vi "Задание_АБ_расп._Рэлея.vi"() -> ()   [LabVIEW 2017]
uses:
  <vilib>/gmath/statdist.llb/Beta Random.vi
  <vilib>/Analysis/3filter.llb/Bessel Filter (DBL).vi
  <vilib>/Analysis/NI_AALBase.lvlib
  <vilib>/gmath/NI_Gmath.lvlib
panel:
  in  "Параметр масштаба":dbl=0.5 format="%#_13g"
  in  "Медиана":dbl=0.1 format="%#_13g"
  out "Шум на основе распределения Рэлея":dbl[](graph)
  out "Итого. кол-во бит":i32
  in  "Пороговое \nзначение":dbl(slide) scale=-0.5..5.0
  out "Демодулированный и отфильтрованный сигнал":dbl[][](graph)
  out "Сигнал после детектора":i16[](graph)
  in  "Нижняя частота среза":dbl
  in  "Порядок фильтра":i64(slide) scale=0.0..20.0
  in  "Переменная floor(x/y)":i32
  out "Модулирующий сигнал":dbl[](graph)
  out "Частотно модулированный цифровой сигнал":dbl[](graph)
  in  "см. 1.2 Циклов в секунду":i32(slide) scale=4.0..50.0
  in  "Сколько битов брать":i32=4
  out "Радио сигнал с паузами":dbl[](graph)
  in  "Кол-во выборок":i32=400
  out "Массив с паузами":dbl[](array[numeric])
  in  "Количество бит":i32=8
  out "Вырезка из массива":dbl[](array[numeric])
  out "Биты на выходе 1":dbl[](array[numeric])
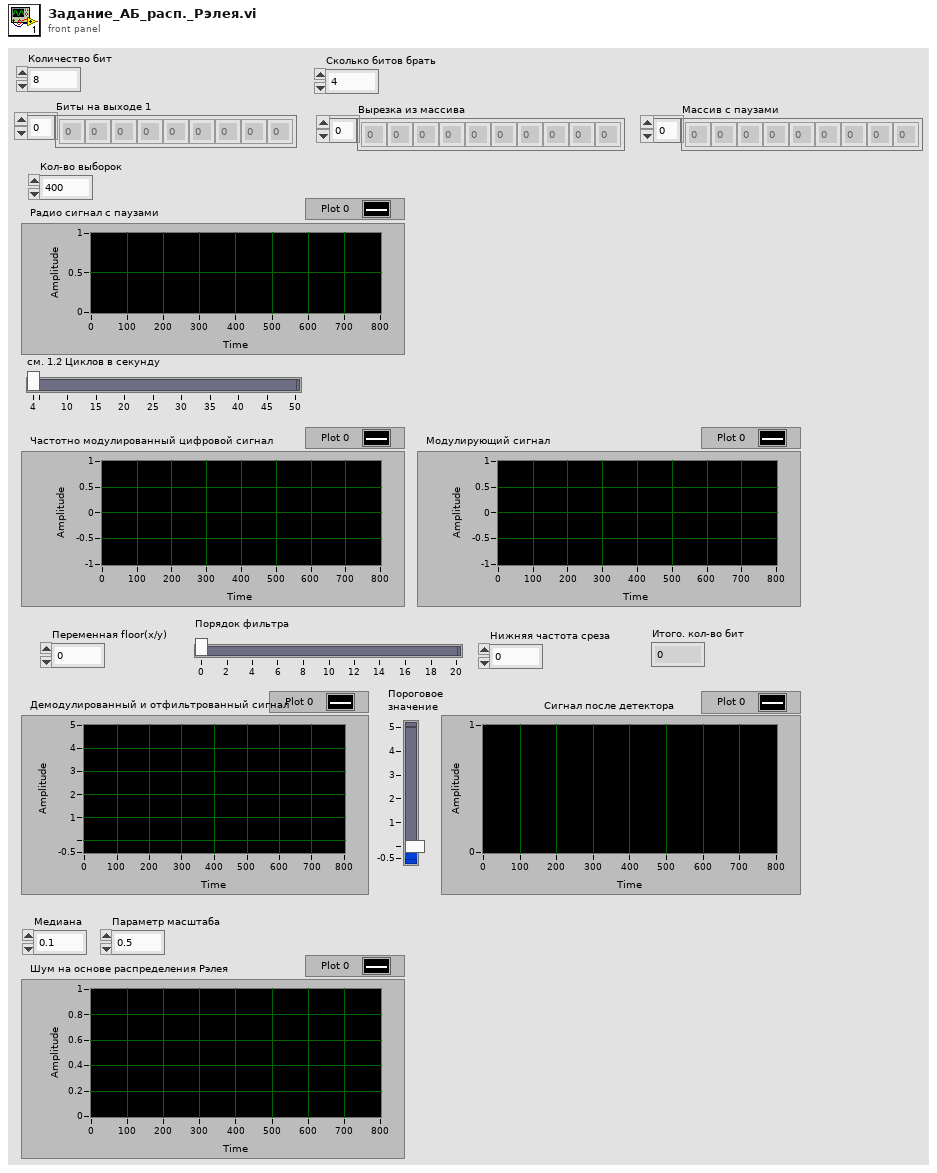
[diagram p1: front panel]
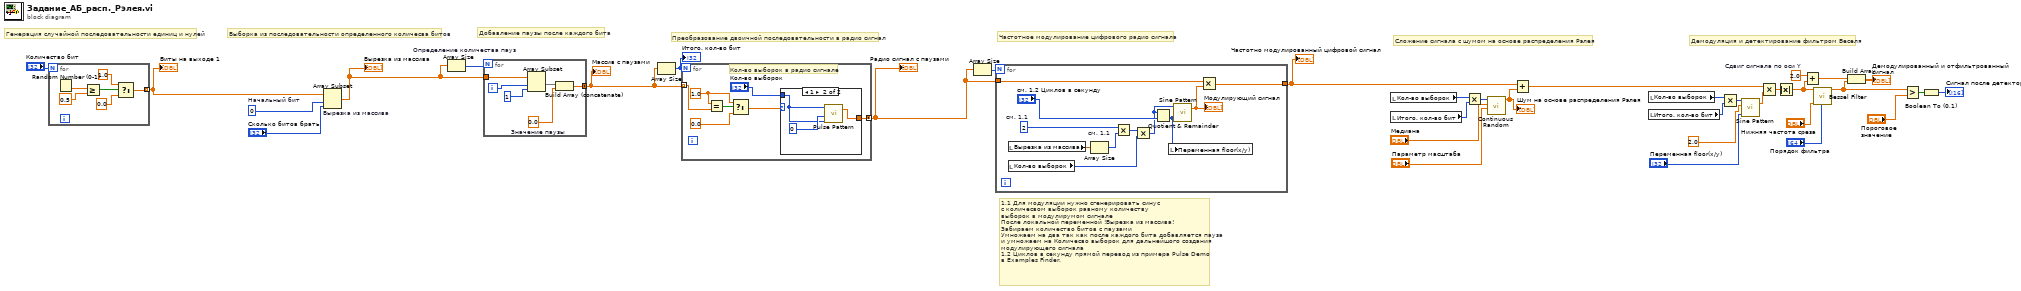
[diagram p0: block diagram]
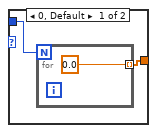
[diagram p2: hidden frame]
diagram:
  w4 = 2.0  # Сдвиг сигнала по оси Y
  w34 = 0  # Начальный бит
  # "Демодуляция и детектирование фильтром Беселя"
  # "Сложение сигнала с шумом на основе распределения Рэлея"
  # "1.1 Для модуляции нужно сгенерировать синус \nс количесвом выборок равному количеству \nвыборок в модулирумом сигнале\nПосле локальной переменной !Вырезка из массива! \nЗабираем количество битов с паузами \nУмножаем на два так как после каждого бита добавляется пауза\nи умножаем на Количесво выборок для дальнейшого создания  \nмодулирующего сигнала\n1.2 Циклов в секунду прямой перевод из примера Pulse Demo \nв Examples Finder."
  # "Преобразование двоичной последовательности в радио сигнал"
  # "Частотное модулирование цифрового радио сигнала"
  # "Добавление паузы после каждого бита"
  # "Выборка из последовательности определенного количесва битов"
  # "Генерация случайной последовательности единиц и нулей"
  n1 = for {
    N: "Количество бит" -> [_]
    tunnel: [w36] -> w32 mode=indexing
    n2 = Random Number (0-1)() -> (number: 0 to 1=w41:dbl)
    n3 = Greater Or Equal?(x=w41, y=0.5) -> (x >= y?=w39:bool)
    n4 = Select(t=1.0, s=w39, f=0.0) -> (s? t:f=w36:dbl)
  }
  "Биты на выходе 1" <- w32
  n5 = Array Subset "Вырезка из массива"(array=w32, index=w34, length="Сколько битов брать") -> (w30:dbl[])
  "Вырезка из массива" <- w30
  n6 = Array Size "Определение количества пауз"(array=w30) -> (size(s)=w31:i32)
  n7 = for {
    N: w31 -> [_]
    tunnel: w30 -> [w44]
    tunnel: [w43] -> w27 mode=concatenating
    i -> [w42]
    w45 = 0.0  # Значение паузы
    n8 = Array Subset(array=w44, index=w42, length=1) -> (w46:dbl[])
    n9 = Build Array (concatenate)(w46, w45) -> (w43:dbl[])
  }
  "Массив с паузами" <- w27
  n10 = Array Size(array=w27) -> (size(s)=w28:i32)
  "Итого. кол-во бит" <- w28
  n11 = for {
    N: w28 -> [_]
    tunnel: w27 -> [w51] mode=indexing
    tunnel: [w49] -> w26 mode=concatenating
    w53 = 1.0
    # "Кол-во выборок в радио сигнале"
    n12 = Equal?(x=w53, y=w51) -> (x = y?=w54:bool)
    n13 = Select(t=w53, s=w54, f=0.0) -> (s? t:f=w50:dbl)
    n14 = case shown="1" w50 {
      tunnel: [w55 w59] -> w49
      tunnel: "Кол-во выборок" -> [w56 w58]
      frame 0, Default {
        n15 = for {
          N: w56 -> [_]
          tunnel: [0.0] -> w55 mode=indexing
        }
      }
      frame 1 {
        n16 = call <vilib>:"Pulse Pattern.vi"("width"=w58, "delay"=0, "samples"=w58) -> ("Pulse Pattern"=w59:dbl[])  [unwired: 1 in, 1 out]
      }
    }
  }
  "Радио сигнал с паузами" <- w26
  n17 = Array Size(array=w26) -> (size(s)=w29:i32)
  n18 = for {
    N: w29 -> [_]
    tunnel: w26 -> [w70]
    tunnel: [w69] -> w8
    w65 = 2  # см. 1.1
    n19 = local read "Вырезка из массива"() -> (w67:dbl[])
    n20 = local read "Кол-во выборок"() -> (w63:i32)
    n21 = Array Size "см. 1.1"(array=w67) -> (size(s)=w66:i32)
    n22 = Multiply(x=w65, y=w66) -> (x*y=w64:i32)
    n23 = Multiply(x=w64, y=w63) -> (x*y=w62:i32)
    n24 = Quotient & Remainder(x=w62, y="см. 1.2 Циклов в секунду") -> (floor(x/y)=w61:i32)  [unwired: 1 out]
    n25 = local write "Переменная floor(x/y)"(w61) -> ()
    n26 = call <vilib>:"Sine Pattern.vi"("cycles"=w61, "samples"=w62) -> ("Sinusoidal Pattern"=w68:dbl[])  [unwired: 2 in, 1 out]
    "Модулирующий сигнал" <- w68
    n27 = Multiply(x=w70, y=w68) -> (x*y=w69:dbl[])
  }
  "Частотно модулированный цифровой сигнал" <- w8
  n28 = local read "Кол-во выборок"() -> (w12:i32)
  n29 = local read "Итого. кол-во бит"() -> (w11:i32)
  n30 = Multiply(x=w12, y=w11) -> (x*y=w10:i32)
  n31 = call-poly <vilib>:"Continuous Random.vi"("b"="Параметр масштаба", "a"="Медиана", "samples"=w10) -> ("beta random data"=w9:dbl[])  [unwired: 7 in, 1 out]
  "Шум на основе распределения Рэлея" <- w9
  n32 = Add(x=w8, y=w9) -> (x+y=w7:dbl[])
  n33 = local read "Кол-во выборок"() -> (w16:i32)
  n34 = local read "Итого. кол-во бит"() -> (w15:i32)
  n35 = Multiply(x=w16, y=w15) -> (x*y=w17:i32)
  n36 = call <vilib>:"Sine Pattern.vi"("cycles"="Переменная floor(x/y)", "amplitude"=2.0, "samples"=w17) -> ("Sinusoidal Pattern"=w18:dbl[])  [unwired: 1 in, 1 out]
  n37 = Multiply(x=w7, y=w18) -> (x*y=w24:dbl[])
  n38 = Absolute Value(x=w24) -> (abs(x)=w2:dbl[])
  n39 = Add(x=w4, y=w2) -> (x+y=w3:dbl[])
  n40 = call-poly <vilib>:"Bessel Filter.vi"("order"="Порядок фильтра", "low cutoff freq: fl"="Нижняя частота среза", "X"=w2) -> ("Filtered X"=w1:dbl[])  [unwired: 5 in, 1 out]
  n41 = Build Array(w3, w1) -> (→"Демодулированный и отфильтрованный сигнал":dbl[][])
  n42 = Greater?(x=w1, y="Пороговое \nзначение") -> (0:w21:bool[])
  n43 = Boolean To (0,1)(Boolean=w21) -> (0, 1=→"Сигнал после детектора":i16[])
